vi "Get and Decode BTI Activity Error and Command Word.vi"(8 "error in":errorcluster, 10 "message fields":T1 {"data" format="%x"; "extra" format="%x"; "msgopt" format="%04x"; "msgflag" format="%04x"; "bus" items=["BUSA", "BUSB", "BUSNONE"]; "cwd1" format="%04x"; "cwd2" format="%04x"; "swd1" format="%04x"; "swd2" format="%04x"}, 11 "map of messages to value indexes":T3) -> (0 "error out":errorcluster, 2 "message fields out":T1 {"data" format="%x"; "extra" format="%x"; "msgopt" format="%04x"; "msgflag" format="%04x"; "bus" items=["BUSA", "BUSB", "BUSNONE"]; "cwd1" format="%04x"; "cwd2" format="%04x"; "swd1" format="%04x"; "swd2" format="%04x"}, 3 "value":T5, 4 "status error counts":T2, 5 "update values":bool)   [LabVIEW 2020, in "AIM MIL-STD-1553 Engine.lvlib" / "Implementation.lvlib" / "Rx Execution Unit.lvclass"]
uses:
  Rx Execution Unit.lvclass
  <instrlib>/BTI1553Lib/BTI1553LV.lvlib
  Shared/Message Map Key.ctl
  Status Error Counts.ctl
  Shared/Address.ctl
  Shared/Terminal Endpoint.ctl
  Shared/Parameter Definition.ctl
  Shared/Message Type.ctl
  Shared/Message Definition.ctl
  Message Map Value.ctl
  Shared/Map of Messages to Value Indexes.ctl
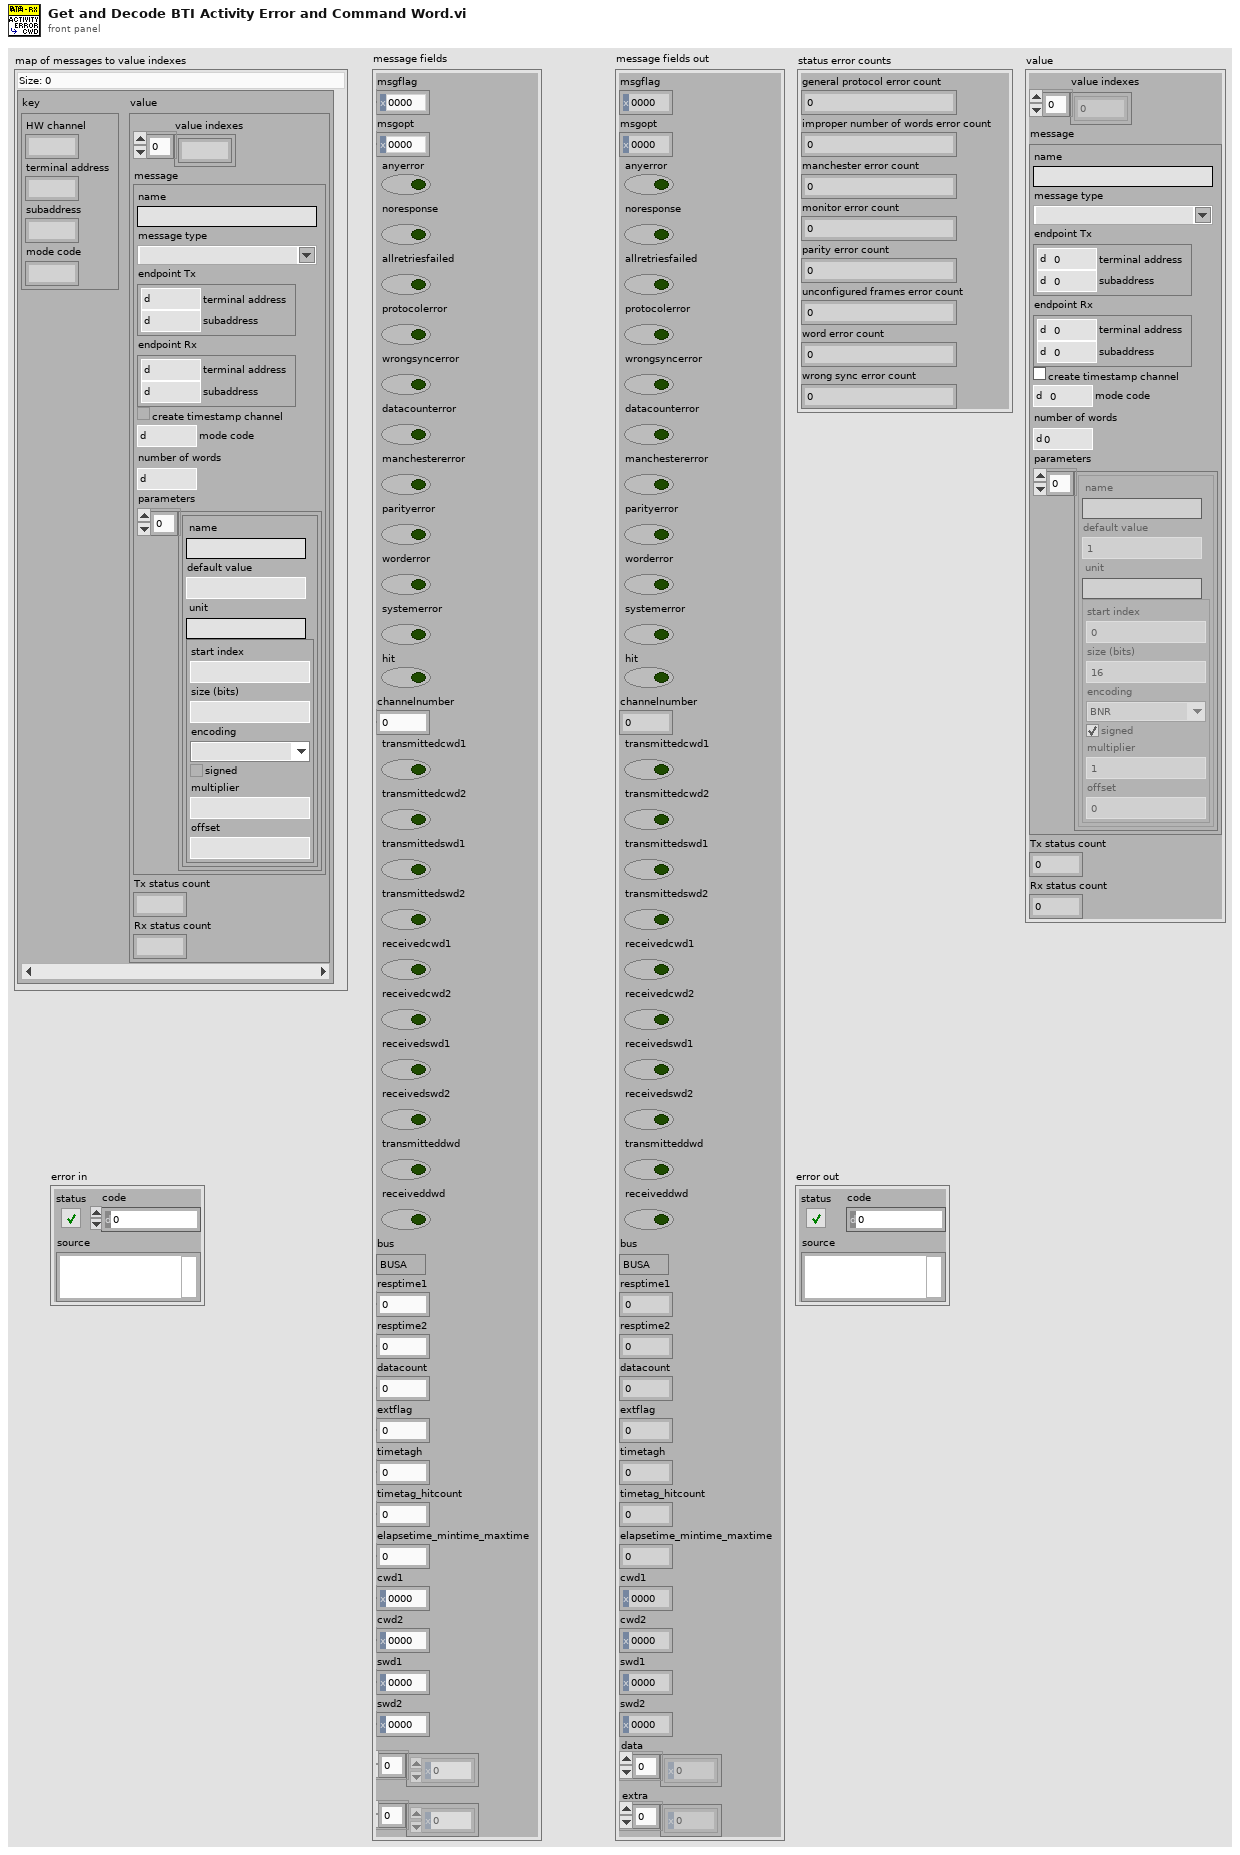
[diagram p1: front panel]
types:
  T1 = cluster{"msgflag":u16, "msgopt":u16, "anyerror":bool, "noresponse":bool, "allretriesfailed":bool, "protocolerror":bool, "wrongsyncerror":bool, "datacounterror":bool, "manchestererror":bool, "parityerror":bool, "worderror":bool, "systemerror":bool, "hit":bool, "reserved":u8, "channelnumber":i32, "transmittedcwd1":bool, "transmittedcwd2":bool, "transmittedswd1":bool, "transmittedswd2":bool, "receivedcwd1":bool, "receivedcwd2":bool, "receivedswd1":bool, "receivedswd2":bool, "transmitteddwd":bool, "receiveddwd":bool, "reserved":i8, "reserved":i8, "bus":u32, "resptime1":u16, "resptime2":u16, "datacount":u16, "extflag":u16, "timetagh":u32, "timetag_hitcount":u32, "elapsetime_mintime_maxtime":u32, "cwd1":u16, "cwd2":u16, "swd1":u16, "swd2":u16, "data":u16[], "extra":u16[]}
  T2 = typedef "AIM MIL-STD-1553 Engine.lvlib/Implementation.lvlib/Rx Execution Unit.lvclass/Status Error Counts.ctl" = cluster{"general protocol error count":u64, "improper number of words error count":u64, "manchester error count":u64, "monitor error count":u64, "parity error count":u64, "unconfigured frames error count":u64, "word error count":u64, "wrong sync error count":u64}
  T3 = typedef "Map of Messages to Value Indexes.ctl" = map{T4, T5}
  T4 = typedef "Message Map Key.ctl" = cluster{"HW channel":u16, "terminal address":u16, "subaddress":u16, "mode code":u16}
  T5 = typedef "AIM MIL-STD-1553 Engine.lvlib/Implementation.lvlib/Rx Execution Unit.lvclass/Message Map Value.ctl" = cluster{"value indexes":i32[], "message":T6, "Tx status count":i32, "Rx status count":i32}
  T6 = typedef "Message Definition.ctl" = cluster{"name":string, "message type":T7, "endpoint Tx":T8, "endpoint Rx":T8, "create timestamp channel":bool, "mode code":u16, "number of words":u16, "parameters":cluster{"name":string, "default value":dbl, "unit":string, "parameter definition":T10}[]}
  T7 = typedef "Message Type.ctl" = string
  T8 = typedef "Terminal Endpoint.ctl" = cluster{"terminal address":T9, "subaddress":T9}
  T9 = typedef "Address.ctl" = u16
  T10 = typedef "Parameter Definition.ctl" = cluster{"start index":i32, "size (bits)":i32, "encoding":enum16{"BNR", "BCD", "Discrete"}, "signed":bool, "multiplier":dbl, "offset":dbl}
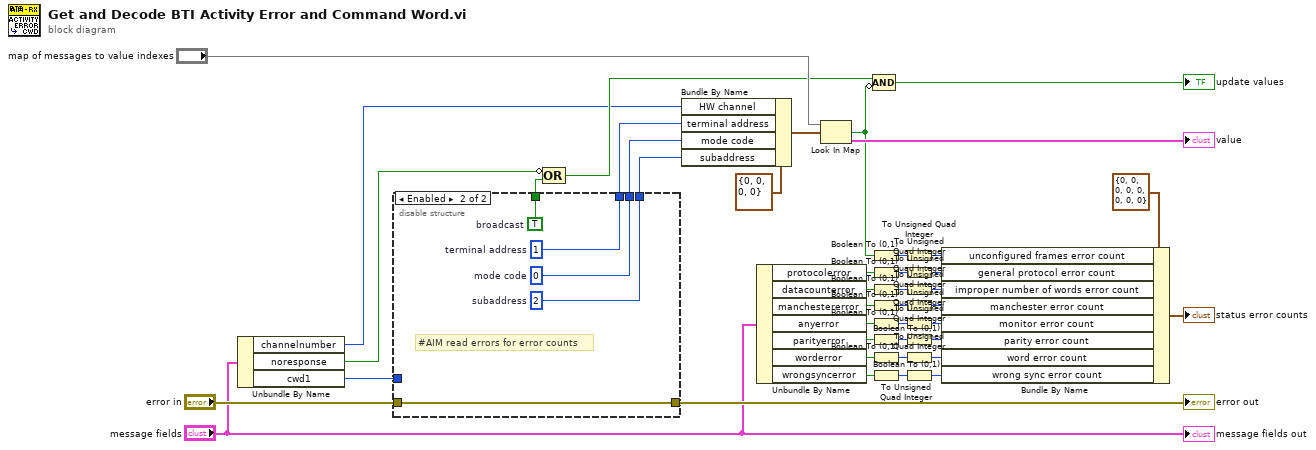
[diagram p0: block diagram]
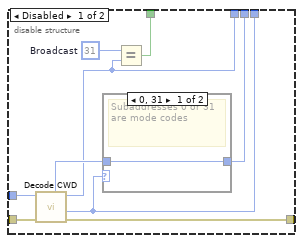
[diagram p2: hidden frame]
diagram:
  n1 = Unbundle By Name("message fields") -> ("channelnumber"=w6:i32, "noresponse"=w7:bool, "cwd1"=w30:u16)
  n2 = disable-structure shown="Enabled" {
    disable-tunnel: [w51 w56] -> w40
    disable-tunnel: [w50 w57] -> w39
    disable-tunnel: "error in" -> [w47 w57]
    disable-tunnel: w30 -> [w46 _]
    disable-tunnel: [w45 w53] -> w5
    disable-tunnel: [w44 w54] -> w4
    disable-tunnel: [w43 w55] -> w2
    frame Disabled {
      w48 = 31  # Broadcast
      n3 = call <instrlib>:"Decode CWD.vi"("error in (no error)"=w47, "command word"=w46) -> ("error out"=w50:errorcluster, "subaddress out"=w45:i32, "terminal address out"=w43:i32, "word count out"=w49:i32)  [unwired: 5 in, 1 out]
      n4 = case shown="0, 31" w45 {
        tunnel: w49 -> [w52 _]
        tunnel: [w52 _] -> w44
        frame 0, 31 {
          # "Subaddresses 0 or 31 are mode codes"
        }
        frame Default {
        }
      }
      n5 = Equal?(x=w48, y=w43) -> (x = y?=w51:bool)
    }
    frame Enabled {
      w53 = 2  # subaddress
      w54 = 0  # mode code
      w55 = 1  # terminal address
      w56 = TRUE  # broadcast
      # "#AIM read errors for error counts"
    }
  }
  "error out" <- w39
  n6 = Compound Arithmetic op=OR(invert w7, w40) -> (w32:bool)
  n7 = Bundle By Name(cluster=T4 {"HW channel"=0, "terminal address"=0, "subaddress"=0, "mode code"=0} ("key"), "HW channel"=w6, "terminal address"=w2, "mode code"=w4, "subaddress"=w5) -> (w42:T4)
  n8 = Unbundle By Name("message fields") -> ("protocolerror"=w26:bool, "datacounterror"=w25:bool, "manchestererror"=w24:bool, "anyerror"=w18:bool, "parityerror"=w19:bool, "worderror"=w21:bool, "wrongsyncerror"=w20:bool)
  n9 = Look In Map(map="map of messages to value indexes", key=w42) -> (key not found?=w3:bool, value=→"value":T5)  [unwired: 1 in]
  n10 = Boolean To (0,1)(Boolean=w3) -> (0, 1=w36:i16)
  n11 = Boolean To (0,1)(Boolean=w26) -> (0, 1=w28:i16)
  n12 = Boolean To (0,1)(Boolean=w25) -> (0, 1=w23:i16)
  n13 = Boolean To (0,1)(Boolean=w24) -> (0, 1=w17:i16)
  n14 = Boolean To (0,1)(Boolean=w18) -> (0, 1=w16:i16)
  n15 = Boolean To (0,1)(Boolean=w19) -> (0, 1=w15:i16)
  n16 = Boolean To (0,1)(Boolean=w21) -> (0, 1=w14:i16)
  n17 = Boolean To (0,1)(Boolean=w20) -> (0, 1=w13:i16)
  n18 = Compound Arithmetic op=AND(w32, invert w3) -> (→"update values":bool)
  n19 = To Unsigned Quad Integer(1:w36) -> (0:w35:u64)
  n20 = To Unsigned Quad Integer(1:w28) -> (0:w27:u64)
  n21 = To Unsigned Quad Integer(1:w23) -> (0:w22:u64)
  n22 = To Unsigned Quad Integer(1:w17) -> (0:w8:u64)
  n23 = To Unsigned Quad Integer(1:w16) -> (0:w9:u64)
  n24 = To Unsigned Quad Integer(1:w15) -> (0:w10:u64)
  n25 = To Unsigned Quad Integer(1:w14) -> (0:w11:u64)
  n26 = To Unsigned Quad Integer(1:w13) -> (0:w12:u64)
  n27 = Bundle By Name(cluster=T2 {"general protocol error count"=0, "improper number of words error count"=0, "manchester error count"=0, "monitor error count"=0, "parity error count"=0, "unconfigured frames error count"=0, "word error count"=0, "wrong sync error count"=0} ("status error counts"), "unconfigured frames error count"=w35, "general protocol error count"=w27, "improper number of words error count"=w22, "manchester error count"=w8, "monitor error count"=w9, "parity error count"=w10, "word error count"=w11, "wrong sync error count"=w12) -> (→"status error counts":T2)
  "message fields out" <- "message fields"
